vi "sub_wattstodBmconversion.vi"(10 "Amp or Power":i32=20, 11 "detected amplitude":dbl) -> (3 "Numeric":dbl)   [LabVIEW 2021]
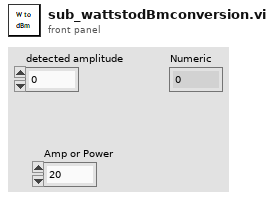
[diagram p1: front panel]
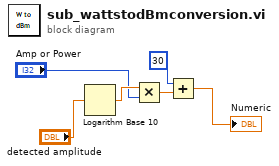
[diagram p0: block diagram]
diagram:
  n1 = Logarithm Base 10(1:"detected amplitude") -> (0:w2:dbl)
  n2 = Multiply(x=w2, y="Amp or Power") -> (x*y=w4:dbl)
  n3 = Add(x=30, y=w4) -> (x+y=→"Numeric":dbl)
